vi "Path Is Funnel.vi"(1 "Path Information":T2) -> (0 "Is Funnel?":bool)   [LabVIEW 2019]
doc: "This VI determines whether or not a path is actually a funnel. It must have two curves (C's) and if it has a line (L), the last point must be the same as the starting point."
uses:
  <vilib>/Analysis/Matrix/Datatypes/RealMatrix.ctl
  Classes/Tool/Tool Data/Tool Data/Tool Data.lvclass
  <vilib>/Analysis/Matrix/NI_Matrix.lvlib
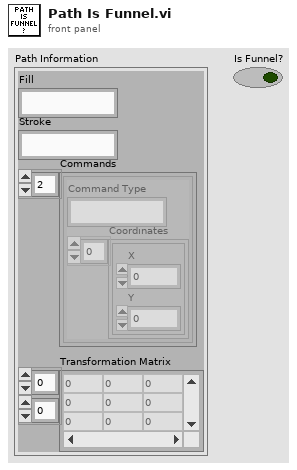
[diagram p1: front panel]
types:
  T1 = typedef "NI_Matrix.lvlib/RealMatrix.ctl" = dbl[][]
  T2 = cluster{"Fill":string, "Stroke":string, "Commands":cluster{"Command Type":string, "Coordinates":cluster{"X":dbl, "Y":dbl}[]}[], "Transformation Matrix":T1}
  T3 = cluster{"Command Type":string, "Coordinates":cluster{"X":dbl, "Y":dbl}[]}[]
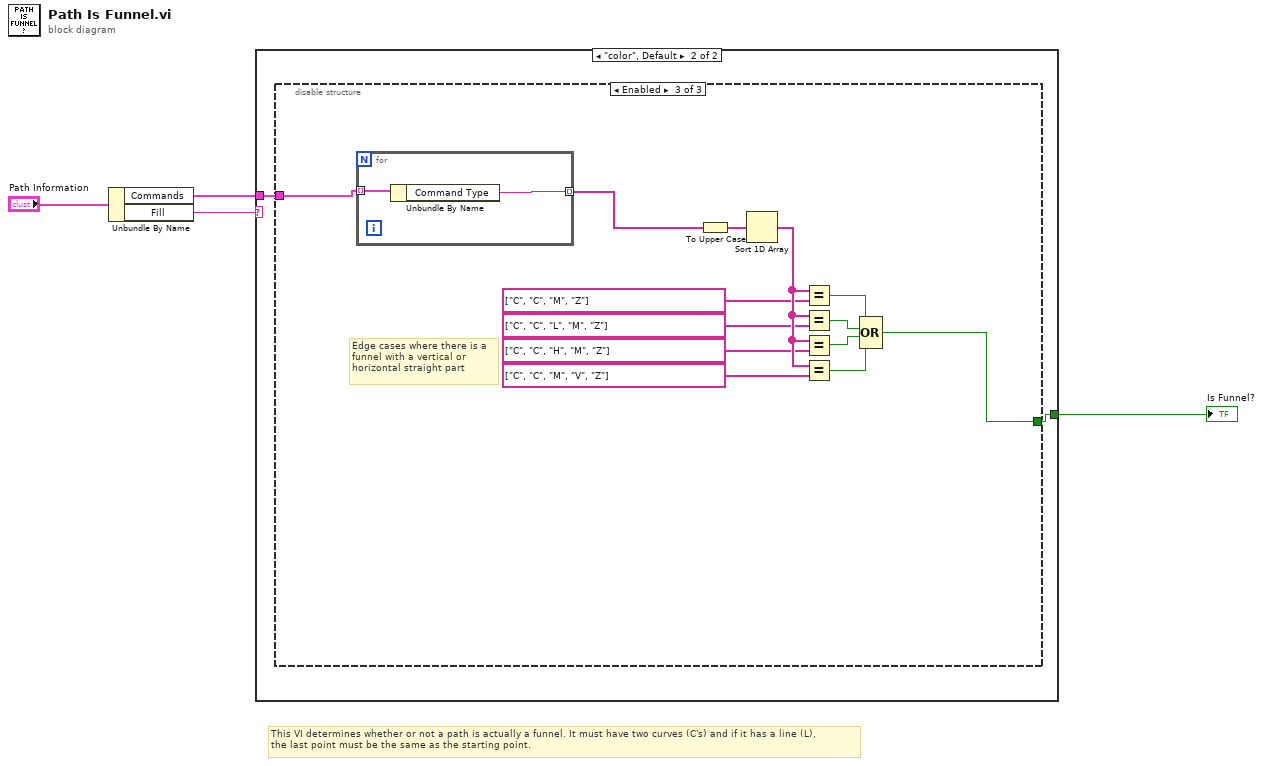
[diagram p0: block diagram]
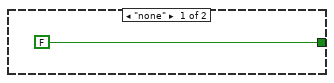
[diagram p2: hidden frame]
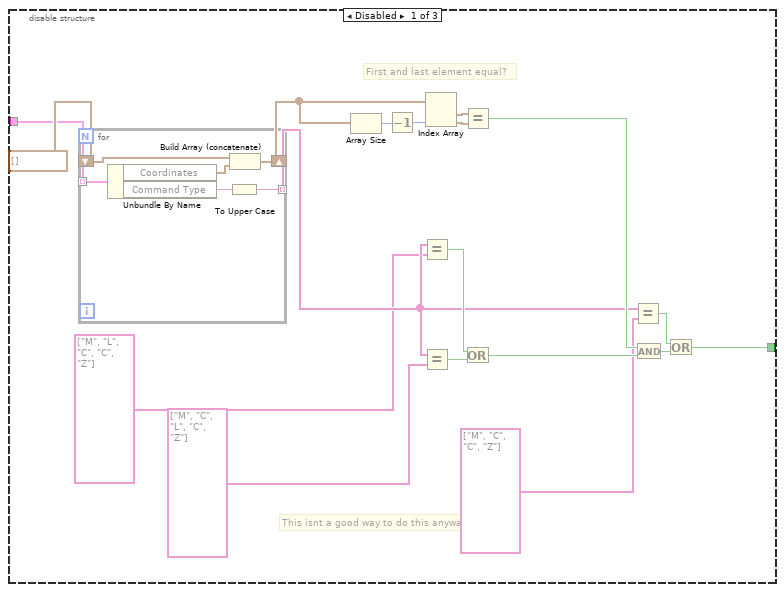
[diagram p3: hidden frame]
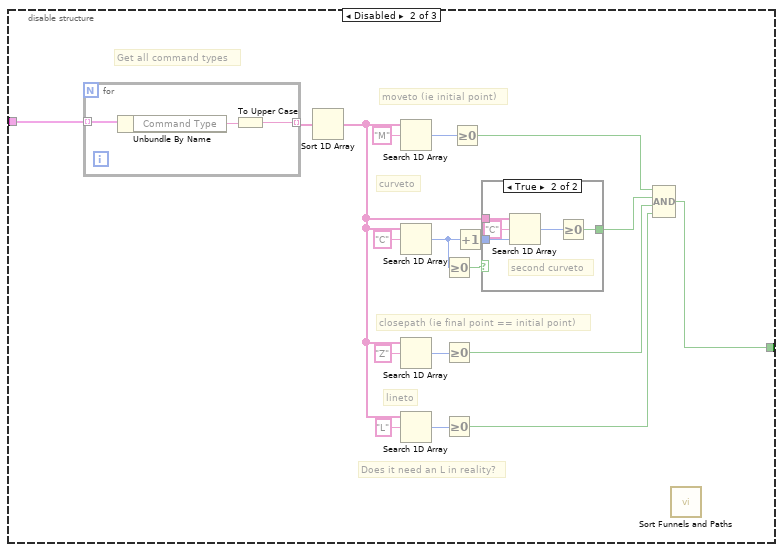
[diagram p4: hidden frame]
diagram:
  # "This VI determines whether or not a path is actually a funnel. It must have two curves (C's) and if it has a line (L),\nthe last point must be the same as the starting point."
  n1 = Unbundle By Name("Path Information") -> ("Commands"=w3:T3, "Fill"=w4:string)
  n2 = case shown="\"color\", Default" w4 {
    tunnel: w3 -> [_ w7]
    tunnel: [FALSE w6] -> w1
    frame "none" {
    }
    frame "color", Default {
      n3 = disable-structure shown="Enabled" {
        disable-tunnel: w7 -> [w10 w49 w61]
        disable-tunnel: [w9 w47 w59] -> w6
        frame Disabled {
          # "This isnt a good way to do this anyways"
          # "First and last element equal?"
          n4 = for {
            tunnel: w10 -> [w31] mode=indexing
            tunnel: [w26] -> w11 mode=indexing
            shift-right: [w29] -> w16
            shift-left: cluster{"X":dbl, "Y":dbl}[] [] -> [w30]
            n5 = Unbundle By Name(w31) -> ("Coordinates"=w28:cluster{"X":dbl, "Y":dbl}[], "Command Type"=w27:string)
            n6 = To Upper Case(1:w27) -> (0:w26:string)
            n7 = Build Array (concatenate)(w30, w28) -> (w29:cluster{"X":dbl, "Y":dbl}[])
          }
          n8 = Array Size(array=w16) -> (size(s)=w15:i32)
          n9 = Decrement(x=w15) -> (x-1=w14:i32)
          n10 = Equal?(x=w11, y=string[] ["M", "L", "C", "C", "Z"]) -> (x = y?=w18:bool)
          n11 = Equal?(x=w11, y=string[] ["M", "C", "L", "C", "Z"]) -> (x = y?=w17:bool)
          n12 = Index Array(array=w16, index #2=w14) -> (element #1=w21:cluster{"X":dbl, "Y":dbl}, element #2=w22:cluster{"X":dbl, "Y":dbl})  [unwired: 1 in]
          n13 = Equal?(x=w21, y=w22) -> (x = y?=w23:bool)
          n14 = Or(x=w18, y=w17) -> (x .or. y?=w20:bool)
          n15 = Equal?(x=w11, y=string[] ["M", "C", "C", "Z"]) -> (x = y?=w25:bool)
          n16 = And(x=w23, y=w20) -> (x .and. y?=w24:bool)
          n17 = Or(x=w25, y=w24) -> (x .or. y?=w9:bool)
        }
        frame Disabled {
          # "Does it need an L in reality?"
          # "lineto"
          # "closepath (ie final point == initial point)"
          # "curveto"
          # "moveto (ie initial point)"
          # "Get all command types"
          n18 = for {
            tunnel: w49 -> [w58] mode=indexing
            tunnel: [w56] -> w48 mode=indexing
            n19 = Unbundle By Name(w58) -> ("Command Type"=w57:string)
            n20 = To Upper Case(1:w57) -> (0:w56:string)
          }
          n21 = Sort 1D Array(array=w48) -> (sorted array=w32:string[])
          n22 = Search 1D Array(1D array=w32, element="M") -> (index of element=w44:i32)  [unwired: 1 in]
          n23 = Search 1D Array(1D array=w32, element="C") -> (index of element=w43:i32)  [unwired: 1 in]
          n24 = Search 1D Array(1D array=w32, element="Z") -> (index of element=w40:i32)  [unwired: 1 in]
          n25 = Search 1D Array(1D array=w32, element="L") -> (index of element=w35:i32)  [unwired: 1 in]
          n26 = Greater Or Equal To 0?(x=w43) -> (x >= 0?=w42:bool)
          n27 = Greater Or Equal To 0?(x=w40) -> (x >= 0?=w37:bool)
          n28 = Greater Or Equal To 0?(x=w35) -> (x >= 0?=w33:bool)
          n29 = Greater Or Equal To 0?(x=w44) -> (x >= 0?=w39:bool)
          n30 = Increment(x=w43) -> (x+1=w36:i32)
          n31 = case shown="True" w42 {
            selector: w42 -> [w50 _]
            tunnel: w36 -> [_ w55]
            tunnel: w32 -> [_ w54]
            tunnel: [w50 w52] -> w38
            frame False {
            }
            frame True {
              # "second curveto"
              n32 = Search 1D Array(1D array=w54, element="C", start index (0)=w55) -> (index of element=w53:i32)
              n33 = Greater Or Equal To 0?(x=w53) -> (x >= 0?=w52:bool)
            }
          }
          n34 = Compound Arithmetic op=AND(w39, w38, w37, w33) -> (w47:bool)
          n35 = call "Sort Funnels and Paths.vi"() -> ()  [unwired: 10 in, 2 out]
        }
        frame Enabled {
          # "Edge cases where there is a funnel with a vertical or horizontal straight part"
          n36 = for {
            tunnel: w61 -> [w73] mode=indexing
            tunnel: [w72] -> w60 mode=indexing
            n37 = Unbundle By Name(w73) -> ("Command Type"=w72:string)
          }
          n38 = To Upper Case(1:w60) -> (0:w71:string[])
          n39 = Sort 1D Array(array=w71) -> (sorted array=w70:string[])
          n40 = Equal?(x=w70, y=string[] ["C", "C", "M", "Z"] ("sorted array")) -> (x = y?=w69:bool)
          n41 = Equal?(x=w70, y=string[] ["C", "C", "L", "M", "Z"] ("sorted array")) -> (x = y?=w67:bool)
          n42 = Equal?(x=w70, y=string[] ["C", "C", "H", "M", "Z"] ("sorted array")) -> (x = y?=w66:bool)
          n43 = Equal?(x=w70, y=string[] ["C", "C", "M", "V", "Z"] ("sorted array")) -> (x = y?=w68:bool)
          n44 = Compound Arithmetic op=OR(w69, w67, w66, w68) -> (w59:bool)
        }
      }
    }
  }
  "Is Funnel?" <- w1
